vi "FFT_Alpha_Beta_Power_Extractor_all_Channel.vi"(11 "NChan EEG Signal":dbl[][](array[numeric])) -> (2 "Beta_all":dbl[](array[numeric]), 3 "Alpha_all":dbl[](array[numeric]))   [LabVIEW 2014]
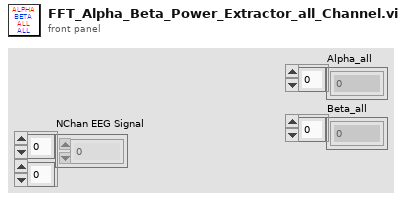
[diagram p1: front panel]
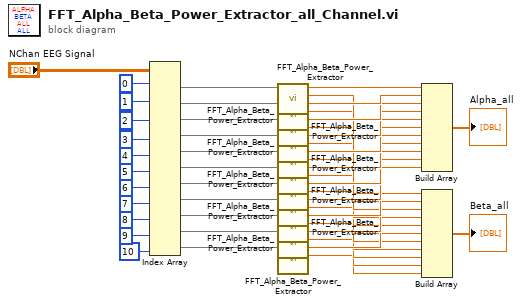
[diagram p0: block diagram]
diagram:
  n1 = Index Array(array="NChan EEG Signal", index (row) #1=0 ("index"), index (row) #2=1 ("index"), index (row) #3=2 ("index"), index (row) #4=3 ("index"), index (row) #5=4 ("index"), index (row) #6=5 ("index"), index (row) #7=6 ("index"), index (row) #8=7 ("index"), index (row) #9=8 ("index"), index (row) #10=9 ("index"), index (row) #11=10 ("index")) -> (element #1=w35:dbl[], element #2=w34:dbl[], element #3=w33:dbl[], element #4=w32:dbl[], element #5=w31:dbl[], element #6=w30:dbl[], element #7=w29:dbl[], element #8=w28:dbl[], element #9=w27:dbl[], element #10=w26:dbl[], element #11=w25:dbl[])  [unwired: 11 in]
  n2 = call "FFT_Alpha_Beta_Power_Extractor.vi"("EEG_Signal"=w35) -> ("Beta"=w13:dbl, "Alpha"=w24:dbl)  [unwired: 9 in]
  n3 = call "FFT_Alpha_Beta_Power_Extractor.vi"("EEG_Signal"=w34) -> ("Beta"=w12:dbl, "Alpha"=w23:dbl)  [unwired: 9 in]
  n4 = call "FFT_Alpha_Beta_Power_Extractor.vi"("EEG_Signal"=w33) -> ("Beta"=w11:dbl, "Alpha"=w22:dbl)  [unwired: 9 in]
  n5 = call "FFT_Alpha_Beta_Power_Extractor.vi"("EEG_Signal"=w32) -> ("Beta"=w10:dbl, "Alpha"=w21:dbl)  [unwired: 9 in]
  n6 = call "FFT_Alpha_Beta_Power_Extractor.vi"("EEG_Signal"=w31) -> ("Beta"=w9:dbl, "Alpha"=w20:dbl)  [unwired: 9 in]
  n7 = call "FFT_Alpha_Beta_Power_Extractor.vi"("EEG_Signal"=w30) -> ("Beta"=w8:dbl, "Alpha"=w19:dbl)  [unwired: 9 in]
  n8 = call "FFT_Alpha_Beta_Power_Extractor.vi"("EEG_Signal"=w29) -> ("Beta"=w7:dbl, "Alpha"=w18:dbl)  [unwired: 9 in]
  n9 = call "FFT_Alpha_Beta_Power_Extractor.vi"("EEG_Signal"=w28) -> ("Beta"=w6:dbl, "Alpha"=w17:dbl)  [unwired: 9 in]
  n10 = call "FFT_Alpha_Beta_Power_Extractor.vi"("EEG_Signal"=w27) -> ("Beta"=w5:dbl, "Alpha"=w16:dbl)  [unwired: 9 in]
  n11 = call "FFT_Alpha_Beta_Power_Extractor.vi"("EEG_Signal"=w26) -> ("Beta"=w4:dbl, "Alpha"=w15:dbl)  [unwired: 9 in]
  n12 = call "FFT_Alpha_Beta_Power_Extractor.vi"("EEG_Signal"=w25) -> ("Beta"=w3:dbl, "Alpha"=w14:dbl)  [unwired: 9 in]
  n13 = Build Array(w24, w23, w22, w21, w20, w19, w18, w17, w16, w15, w14) -> (→"Alpha_all":dbl[])
  n14 = Build Array(w13, w12, w11, w10, w9, w8, w7, w6, w5, w4, w3) -> (→"Beta_all":dbl[])
